vi "Reset Series ROI.vi"(8 "error in (no error)":errorcluster, 11 "Series Graph in":refnum<class "Series Graph.lvclass">) -> (0 "error out":errorcluster, 3 "Series Graph out":refnum<class "Series Graph.lvclass">)   [LabVIEW 2023, in "Series Graph.lvclass"]
uses:
  Series Graph.lvclass
  Series Graph.lvclass/Series Graph.ctl
  Detail Graph/Detail Graph.lvclass
  D:/git/Graph-Classes/Detail Graph/Detail Graph.lvclass
  D:/git/Graph-Classes/Base Graph/Base Graph.lvclass
  D:/git/Graph-Classes/Series Graph/Series Graph.lvclass
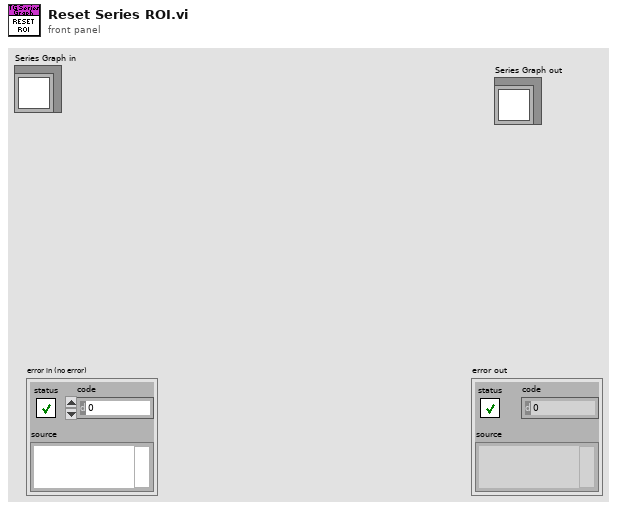
[diagram p1: front panel]
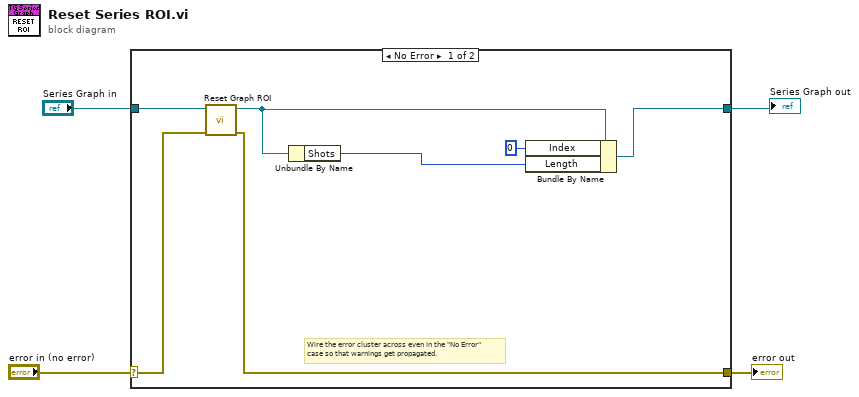
[diagram p0: block diagram]
diagram:
  n1 = case shown="No Error" "error in (no error)" {
    selector: "error in (no error)" -> [w10 w13]
    tunnel: [w5 w13] -> w3
    tunnel: [w8 w12] -> w1
    tunnel: "Series Graph in" -> [w11 w12]
    frame No Error {
      # "Wire the error cluster across even in the \"No Error\"\ncase so that warnings get propagated."
      n2 = call "Reset Graph ROI.vi"("error in (no error)"=w10, "Detail Graph. in"=w11) -> ("error out"=w5:errorcluster, "Detail Graph. out"=w9:refnum<class "Series Graph.lvclass">)  [unwired: 8 in]
      n3 = Unbundle By Name(w9) -> ("Shots"=w6:u32)
      n4 = Bundle By Name(cluster=w9, "Index"=u32 0 ("Z-ROI.Index"), "Length"=w6) -> (w8:refnum<class "Series Graph.lvclass">)
    }
    frame Error {
    }
  }
  "error out" <- w3
  "Series Graph out" <- w1
